vi "Global_CMD_Data Out.vi"() -> ()   [LabVIEW 2020, in "Template_CMD.lvlib"]
uses:
  Template_CMD.lvlib
panel:
  in  "CMD_Template_CycleTime(S)":dbl
  # "The Names of the Data items in the Global Variable MUST describe who the Single Writer is\nFor CMD Globals the the naming convention is\n   \nCMD_Lib Name_Data Name\n\nExamples:\nCMD_RobotArm_Mode\nCMD_AutoTrack_Mode"
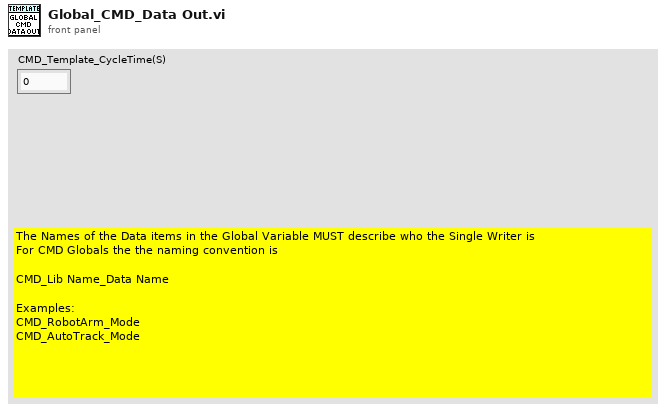
[diagram p1: front panel]
diagram:
